vi "Demo_MAC Address Fetcher getmac.vi"(7 "Match Exactly?":bool, 8 "error in (no error)":errorcluster, 9 "Filter Disconnected":bool, 10 "Filter dashes?":bool, 11 "Specific Connection":string="Ethernet") -> (0 "error out":errorcluster, 1 "Connected Array":string[][](array[string]), 2 "Specific Connection":string[][](array[string]), 3 "First Matched MAC":string, 5 "Full Array":string[][](array[string]))   [LabVIEW 2017]
doc: "This VI calls a Windows shell command that fetches details of the installed Network Interface Cards. It then searches for valid Physical (MAC) Addresses and populates an array. If \"All adapters\" is set to True, then the whole array will be output. otherwise, only the first element will be output, which should correspond to the primary ethernet adapter."
uses:
  <vilib>/regexp/Match Regular Expression.xnode
panel:
  out "Shell Output":string
  # "Network card MAC Address Fetcher"
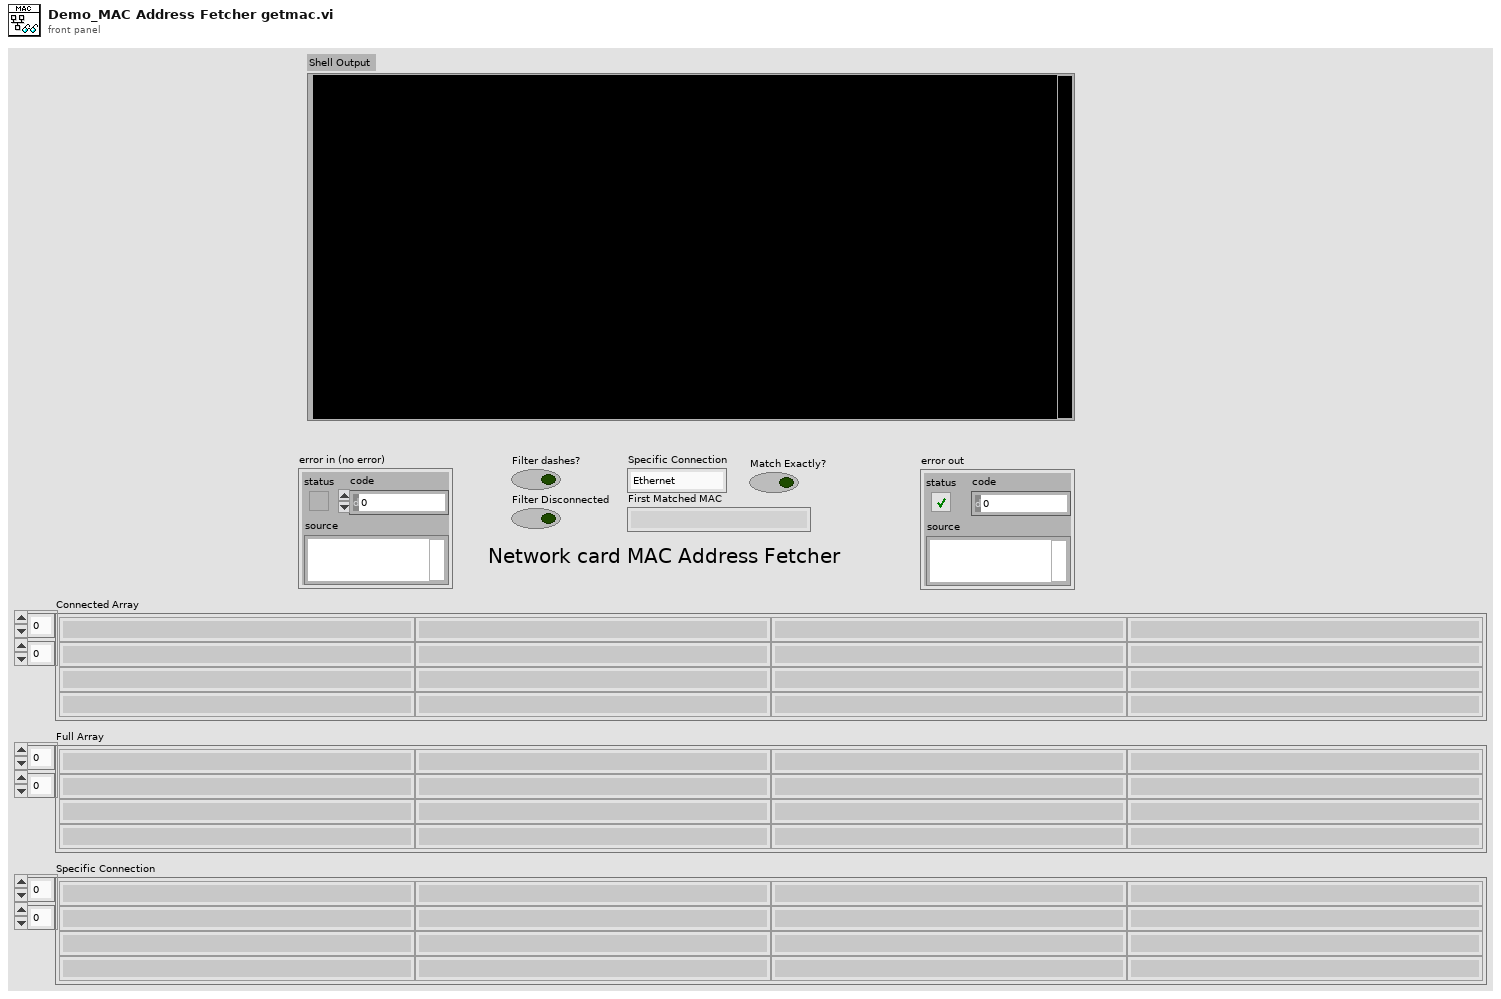
[diagram p1: front panel]
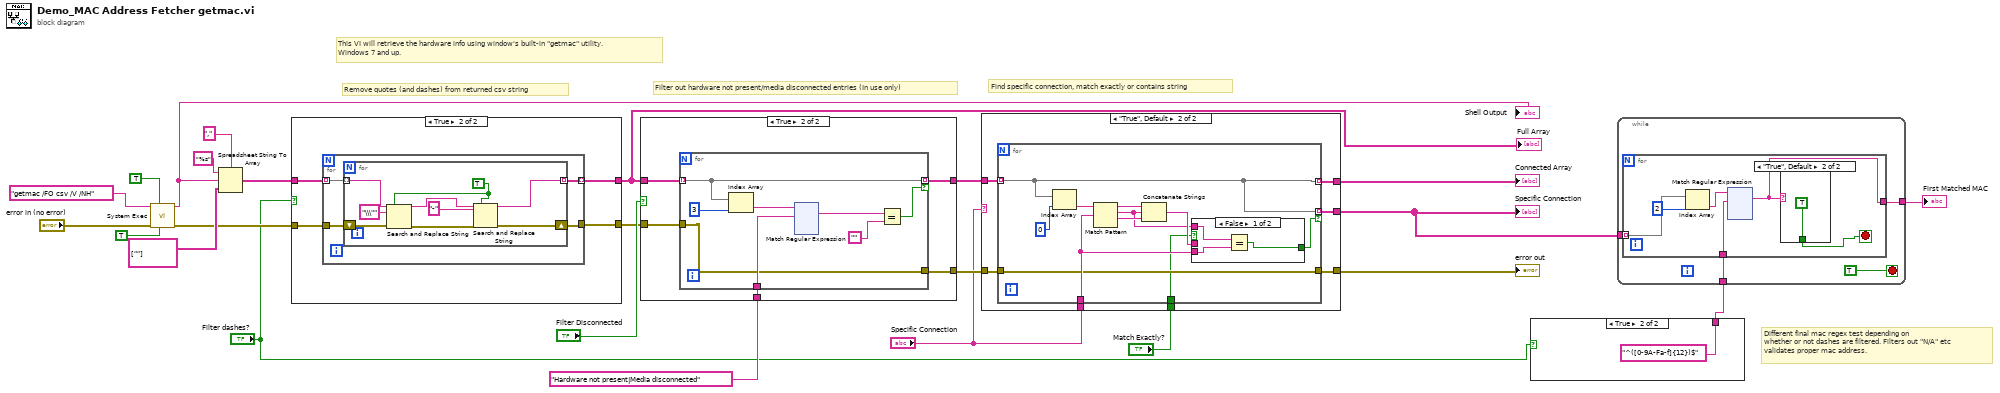
[diagram p0: block diagram]
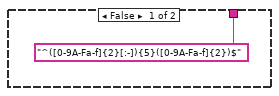
[diagram p2: hidden frame]
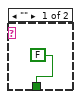
[diagram p3: hidden frame]
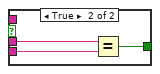
[diagram p5: hidden frame]
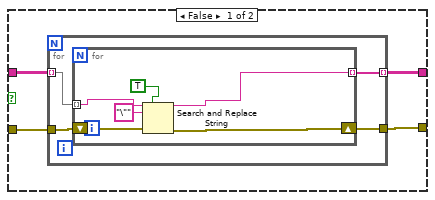
[diagram p7: hidden frame]
diagram:
  # "Different final mac regex test depending on\nwhether or not dashes are filtered. Filters out \"N/A\" etc\nvalidates proper mac address."
  # "Find specific connection, match exactly or contains string"
  # "Filter out hardware not present/media disconnected entries (In use only)"
  # "Remove quotes (and dashes) from returned csv string"
  # "This VI will retrieve the hardware info using window's built-in \"getmac\" utility.\nWindows 7 and up."
  n1 = call <vilib>:"System Exec.vi"("run minimized? (F)"=TRUE, "wait until completion? (T)"=TRUE ("run minimized? (F)"), "error in (no error)"="error in (no error)", "command line"="getmac /FO csv /V /NH") -> ("error out"=w12:errorcluster, "standard output"=w17:string)  [unwired: 4 in, 2 out]
  "Shell Output" <- w17
  n2 = Spreadsheet String To Array(delimiter (Tab)=",", format string="%s", spreadsheet string=w17, array type (2D Dbl)=string[][] [[""]]) -> (array=w13:string[][])
  n3 = case shown="True" "Filter dashes?" {
    tunnel: w12 -> [w28 w40]
    tunnel: [w27 w39] -> w11
    tunnel: w13 -> [w25 w42]
    tunnel: [w26 w41] -> w7
    frame False {
      n4 = for {
        tunnel: w28 -> [w32]
        tunnel: [w31] -> w27
        tunnel: [w29] -> w26 mode=indexing
        tunnel: w25 -> [w30] mode=indexing
        n5 = for {
          tunnel: w30 -> [w36] mode=indexing
          tunnel: [w33] -> w29 mode=indexing
          shift-right: [w34] -> w31
          shift-left: w32 -> [w37]
          n6 = Search and Replace String(replace all?=TRUE, input string=w36, search string="\"", error in=w37) -> (result string=w33:string, error out=w34:errorcluster)  [unwired: 4 in, 2 out]
        }
      }
    }
    frame True {
      n7 = for {
        tunnel: w42 -> [w45] mode=indexing
        tunnel: [w43] -> w41 mode=indexing
        tunnel: w40 -> [w46]
        tunnel: [w44] -> w39
        n8 = for {
          tunnel: w45 -> [w52] mode=indexing
          tunnel: [w48] -> w43 mode=indexing
          shift-right: [w47] -> w44
          shift-left: w46 -> [w54]
          w49 = TRUE ("replace all? (F)")
          n9 = Search and Replace String(replace all?=w49, input string=w52, search string="\\\"", error in=w54) -> (result string=w51:string, error out=w53:errorcluster)  [unwired: 4 in, 2 out]
          n10 = Search and Replace String(replace all?=w49, input string=w51, search string="-", error in=w53) -> (result string=w48:string, error out=w47:errorcluster)  [unwired: 4 in, 2 out]
        }
      }
    }
  }
  "Full Array" <- w7
  n11 = case shown="True" "Filter Disconnected" {
    tunnel: [w57 w61] -> w10
    tunnel: [w56 w58] -> w9
    tunnel: w7 -> [w56 w60]
    tunnel: w11 -> [w57 w62]
    tunnel: "Hardware not present|Media disconnected" -> [_ w59]
    frame False {
    }
    frame True {
      n12 = for {
        tunnel: w62 -> [w63]
        tunnel: w60 -> [w67] mode=indexing
        tunnel: w59 -> [w69]
        tunnel: [w67] -> w58 mode=indexing if=w68
        tunnel: [w63] -> w61
        n13 = Index Array(array=w67, index=3) -> (element=w66:string)
        n14 = xnode "Match Regular Expression"("input string"=w66, "regular expression"=w69) -> ("whole match"=w65:string)  [unwired: 4 in, 4 out]
        n15 = Equal?(x=w65, y="") -> (x = y?=w68:bool)
      }
    }
  }
  n16 = case shown="\"True\", Default" "Specific Connection" {
    tunnel: "Specific Connection" -> [_ w193]
    tunnel: [w186 w192] -> w19
    tunnel: [w186 w191] -> w5
    tunnel: [w185 w190] -> w18
    tunnel: w10 -> [w185 w189]
    tunnel: w9 -> [w186 w188]
    tunnel: "Match Exactly?" -> [_ w187]
    frame "" {
    }
    frame "True", Default {
      n17 = for {
        tunnel: w189 -> [w196]
        tunnel: w188 -> [w200] mode=indexing
        tunnel: w193 -> [w202]
        tunnel: [w200] -> w192 mode=indexing
        tunnel: [w200] -> w191 mode=indexing if=w201
        tunnel: [w196] -> w190
        tunnel: w187 -> [w195]
        n18 = Index Array(array=w200, index=0) -> (element=w203:string)
        n19 = Match Pattern(string=w203, regular expression=w202) -> (before substring=w199:string, match substring=w194:string, after substring=w198:string)  [unwired: 1 in, 1 out]
        n20 = Concatenate Strings(w199, w194, w198) -> (w197:string)
        n21 = case shown="False" w195 {
          tunnel: w202 -> [w206 w210]
          tunnel: [w205 w209] -> w201
          tunnel: w197 -> [_ w208]
          tunnel: w194 -> [w207 _]
          frame False {
            n22 = Equal?(x=w207, y=w206) -> (x = y?=w205:bool)
          }
          frame True {
            n23 = Equal?(x=w208, y=w210) -> (x = y?=w209:bool)
          }
        }
      }
    }
  }
  "Connected Array" <- w19
  "Specific Connection" <- w5
  "error out" <- w18
  n24 = case shown="True" "Filter dashes?" {
    tunnel: ["^([0-9A-Fa-f]{2}[:-]){5}([0-9A-Fa-f]{2})$" ("regular expression") "^([0-9A-Fa-f]{12})$" ("regular expression")] -> w2
    frame False {
    }
    frame True {
    }
  }
  n25 = while {
    tunnel: w5 -> [w216]
    tunnel: [w215] -> w4
    tunnel: w2 -> [w213]
    stop <- TRUE stop-if-true
    n26 = for {
      tunnel: w216 -> [w222] mode=indexing
      tunnel: [w218] -> w215
      tunnel: w213 -> [w217]
      stop <- w219 stop-if-true
      n27 = Index Array(array=w222, index=2 ("disabled index (col)")) -> (element=w220:string)
      n28 = xnode "Match Regular Expression"("input string"=w220, "regular expression"=w217) -> ("whole match"=w218:string)  [unwired: 4 in, 4 out]
      n29 = case shown="\"True\", Default" w218 {
        tunnel: [FALSE TRUE] -> w219
        frame "" {
        }
        frame "True", Default {
        }
      }
    }
  }
  "First Matched MAC" <- w4
